vi "OptimusDrive.vi"   [LabVIEW 2015]
uses:
  Sprocket/lib/Sprocket.lvlib
  Sprocket/src/Action/Action Name.ctl
  Sprocket/src/Refname/Queues.ctl
  Sprocket/src/Refname/Refname to String (Queue).vi
  Drive States.ctl
types:
  T1 = typedef "Drive States.ctl" = enum16{"Teleop", "Auto Straight", "Auto Rotating"}
  T2 = typedef "Sprocket.lvlib/Queues.ctl" = enum16{"Input", "Drive", "Collector", "Shifter", "Wedge"}
  T3 = typedef "Sprocket.lvlib/Action Name.ctl" = enum16{"No Action", "Drive Train Left", "Drive Train Right", "Drive Train Both", "Collector Motor Roll", "Collector Motor Eject", "Collector Motor Stop", "Collector Extend", "Collector Retract", "Shifter High", "Shifter Low", "Collector Motor Stall", "Wedge Roll", "Drive Rotate"}
  T4 = typedef "Sprocket.lvlib/Action.ctl" = cluster{"Name":T3, "Priority":i32, "Data":variant}
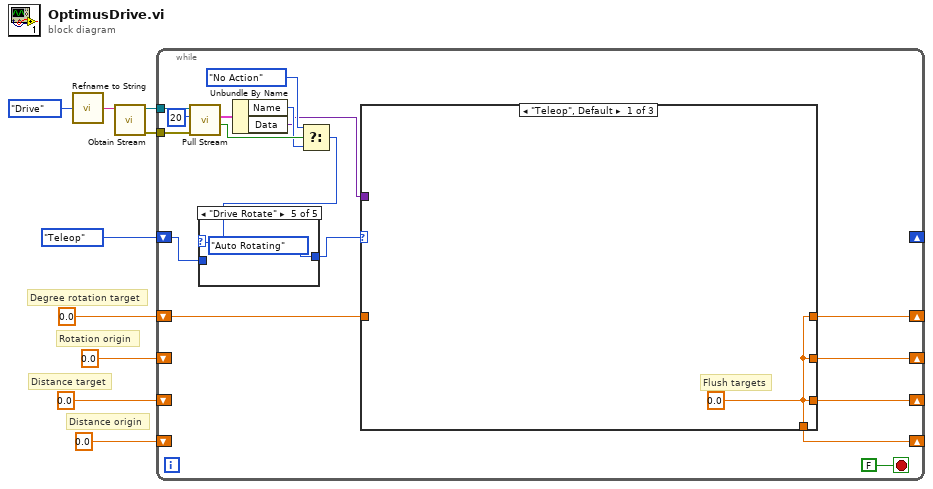
[diagram p0: block diagram]
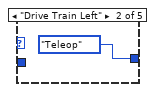
[diagram p3: hidden frame]
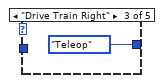
[diagram p4: hidden frame]
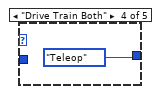
[diagram p5: hidden frame]
diagram:
  # "Distance origin"
  # "Rotation origin"
  # "Distance target"
  # "Degree rotation target"
  n1 = call-poly "Refname to String.vi"("Queue Refname"=Queues."Drive" ("Refname (Queue)")) -> ("Refnum Name"=w9:string)
  n2 = call "Obtain Stream.vi"("Name"=w9) -> ("error out"=w8:errorcluster, "stream out"=w6:refnum<queue>)  [unwired: 9 in]
  n3 = while {
    tunnel: w8 -> [w25]
    tunnel: w6 -> [w24]
    shift-right: _ -> [_]
    shift-left: Drive_States."Teleop" -> [w18]
    shift-right: [w13] -> _
    shift-left: 0.0 -> [w14]
    shift-right: [w11] -> _
    shift-left: 0.0 -> [_]
    shift-right: [w12] -> _
    shift-left: 0.0 -> [_]
    shift-right: [w10] -> _
    shift-left: 0.0 -> [_]
    stop <- FALSE stop-if-true
    n4 = call "Pull Stream.vi"("error in (no error)"=w25, "timeout in ms (-1)"=20, "stream in"=w24) -> ("timed out?"=w23:bool, "element"=w26:T4)  [unwired: 5 in, 2 out]
    n5 = Unbundle By Name(w26) -> ("Name"=w21:T3, "Data"=w15:variant)
    n6 = Select(t=Action_Name."No Action" ("Name"), s=w23, f=w21) -> (s? t:f=w16:T3)
    n7 = case shown="\"Drive Rotate\"" w16 {
      tunnel: w18 -> [w27 _ _ _ _]
      tunnel: [w27 Drive_States."Teleop" Drive_States."Teleop" Drive_States."Teleop" Drive_States."Auto Rotating"] -> w17
      frame "No Action", Default {
      }
      frame "Drive Train Left" {
      }
      frame "Drive Train Right" {
      }
      frame "Drive Train Both" {
      }
      frame "Drive Rotate" {
      }
    }
    n8 = case shown="\"Teleop\", Default" w17 {
      tunnel: w15 -> [_ _ _]
      tunnel: w14 -> [_ _ _]
      tunnel: [w32 _ _] -> w13
      tunnel: [w32 _ _] -> w12
      tunnel: [w32 _ _] -> w11
      tunnel: [w32 _ _] -> w10
      frame "Teleop", Default {
        w32 = 0.0
        # "Flush targets"
      }
      frame "Auto Straight" {
      }
      frame "Auto Rotating" {
      }
    }
  }
